vi "Threshold (SubVI).vi"(7 "Threshold Range":cluster{"Low":u8, "High":u8}, 8 "Input Valid":bool, 11 "Data In":u64) -> (0 "Output Valid":bool, 3 "Data Out":u64)   [LabVIEW 2015]
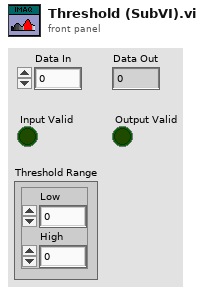
[diagram p1: front panel]
types:
  T1 = cluster{"Numeric Control":u8, "Numeric Control":u8, "Numeric Control":u8, "Numeric Control":u8, "Numeric Control":u8, "Numeric Control":u8, "Numeric Control":u8, "Numeric Control":u8}
  T2 = cluster{"Numeric Control":bool, "Numeric Control":bool, "Numeric Control":bool, "Numeric Control":bool, "Numeric Control":bool, "Numeric Control":bool, "Numeric Control":bool, "Numeric Control":bool}
  T3 = cluster{"Numeric Control":i16, "Numeric Control":i16, "Numeric Control":i16, "Numeric Control":i16, "Numeric Control":i16, "Numeric Control":i16, "Numeric Control":i16, "Numeric Control":i16}
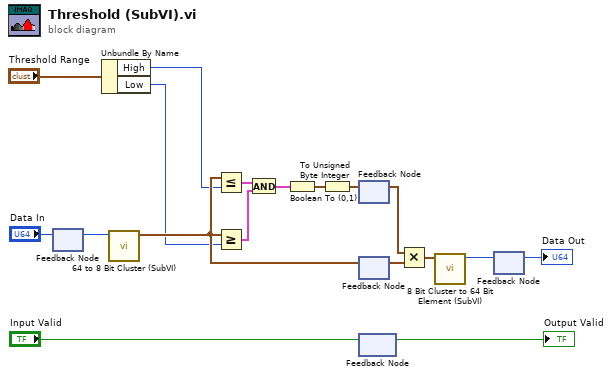
[diagram p0: block diagram]
diagram:
  n1 = feedback #1() -> (w14:u64)  [unwired: 1 in]
  n2 = feedback-in #1("Data In") -> ()
  n3 = Unbundle By Name("Threshold Range") -> ("High"=w2:u8, "Low"=w3:u8)
  n4 = call "64 to 8 Bit Cluster (SubVI).vi"("Data In"=w14) -> ("Data Out"=w8:T1)  [unwired: 10 in]
  n5 = Less Or Equal?(x=w8, y=w2) -> (x <= y?=w4:T2)
  n6 = Greater Or Equal?(x=w8, y=w3) -> (x >= y?=w5:T2)
  n7 = And(x=w4, y=w5) -> (x .and. y?=w6:T2)
  n8 = Boolean To (0,1)(Boolean=w6) -> (0, 1=w7:T3)
  n9 = To Unsigned Byte Integer(number=w7) -> (unsigned 8bit integer=w9:T1)
  n10 = feedback #2() -> (w15:T1)  [unwired: 1 in]
  n11 = feedback-in #2(w9) -> ()
  n12 = feedback #3() -> (w16:T1)  [unwired: 1 in]
  n13 = feedback-in #3(w8) -> ()
  n14 = feedback #4() -> (→"Output Valid":bool)  [unwired: 1 in]
  n15 = feedback-in #4("Input Valid") -> ()
  n16 = Multiply(x=w15, y=w16) -> (x*y=w10:T1)
  n17 = call "8 Bit Cluster to 64 Bit Element (SubVI).vi"("Pixel Cluster"=w10) -> ("Pixel Data (64-Bit)"=w12:u64)  [unwired: 10 in]
  n18 = feedback #5() -> (→"Data Out":u64)  [unwired: 1 in]
  n19 = feedback-in #5(w12) -> ()
